vi "传感器数据.vi"() -> (3 "传感器读数":T1 {"大幅度" format="%#.3f"; "输出扭矩(大)" format="%#.3f"; "大幅" format="%#.3f"; "输入扭矩" format="%#.3f"; "1" format="%#.3f"; "工装移载位移" format="%#.3f"; "电缸位移" format="%#.3f"; "电缸压力" format="%#.3f"})   [LabVIEW 2020]
uses:
  Libraries/S7/S7.lvlib
panel:
  out "单精度浮点":sgl
  out "元素":i32
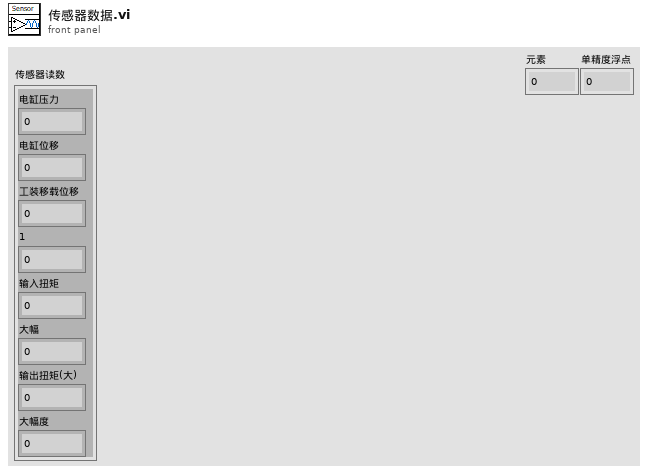
[diagram p1: front panel]
types:
  T1 = cluster{"电缸压力":dbl, "电缸位移":sgl, "工装移载位移":sgl, "1":sgl, "输入扭矩":sgl, "大幅":sgl, "输出扭矩(大)":sgl, "大幅度":sgl}
  T2 = typedef "S7.lvlib/Read_Data (Reply Payload)--cluster.ctl" = cluster{"读取成功":bool, "数据":u32[], "Read_Data_error":errorcluster}
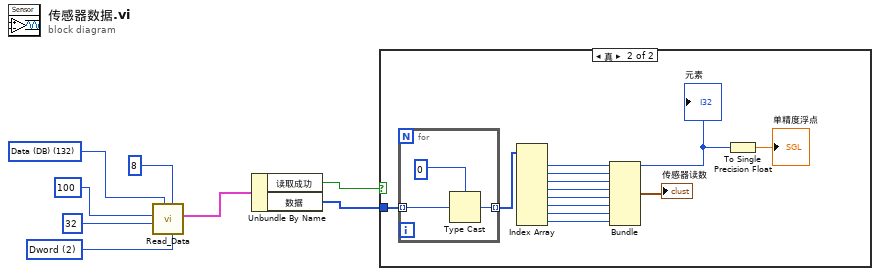
[diagram p0: block diagram]
diagram:
  w5 = u16 2 items=["byte", "word", "Dword"] ("数据类型")
  w6 = u8 132 items=["I/O (P)"=128, "Input (I)"=129, "Output (Q)"=130, "Bit Memory (M)"=131, "Data (DB)"=132, "Instance Data (DI)"=133, "Local Data (L)"=134, "Predecessor Local Data (VL)"=135] ("寄存器类型")
  n1 = call "Read_Data.vi"("数据类型"=w5, "读取长度"=u16 8, "寄存器类型"=w6, "起始地址"=u32 32, "DB #"=u16 100) -> ("Reply Payload"=w3:T2)  [unwired: 4 in, 2 out]
  n2 = Unbundle By Name(w3) -> ("读取成功"=w1:bool, "数据"=w2:u32[])
  n3 = case shown="真" w1 {
    tunnel: w2 -> [_ w20]
    frame False {
    }
    frame True {
      n4 = for {
        tunnel: w20 -> [w23] mode=indexing
        tunnel: [w22] -> w19 mode=indexing
        n5 = Type Cast(type=0, x=w23) -> (*(type *) &x=w22:i32)
      }
      n6 = Index Array(array=w19) -> (element #1=w10:i32, element #2=w18:i32, element #3=w17:i32, element #4=w16:i32, element #5=w14:i32, element #6=w13:i32, element #7=w12:i32, element #8=w15:i32)  [unwired: 8 in]
      "元素" <- w10
      n7 = Bundle(w10, w18, w17, w16, w14, w13, w12, w15) -> (→"传感器读数":cluster{i32, i32, i32, i32, i32, i32, i32, i32})  [unwired: 1 in]
      n8 = To Single Precision Float(number=w10) -> (single precision float=→"单精度浮点":sgl)
    }
  }
